vi "Ways to Win.vi"(11 "Race In":refnum<class "Race.lvclass">) -> (2 "Ways to win":u64, 3 "Race Out":refnum<class "Race.lvclass">)   [LabVIEW 2021, in "Race.lvclass"]
uses:
  Race.lvclass
  Race.lvclass/Race.ctl
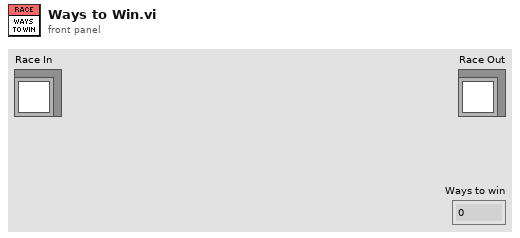
[diagram p1: front panel]
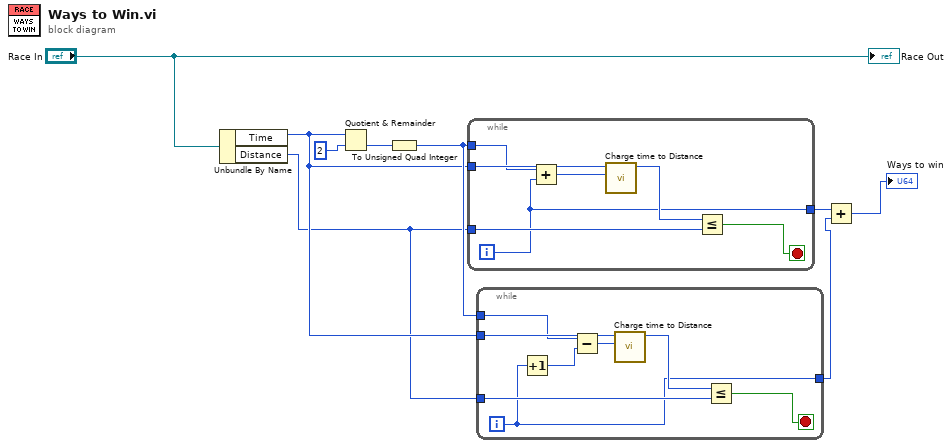
[diagram p0: block diagram]
diagram:
  n1 = Unbundle By Name("Race In") -> ("Time"=w4:u64, "Distance"=w3:u64)
  n2 = Quotient & Remainder(x=w4, y=u64 2) -> (floor(x/y)=w7:u64)  [unwired: 1 out]
  n3 = To Unsigned Quad Integer(1:w7) -> (0:w5:u64)
  n4 = while {
    tunnel: w4 -> [w16]
    tunnel: w5 -> [w15]
    tunnel: w3 -> [w12]
    tunnel: [w10] -> w6
    i -> [w10]
    stop <- w11 stop-if-true
    n5 = Add(x=w15, y=w10) -> (x+y=w14:u64)
    n6 = call "Charge time to Distance.vi"("Charge Time"=w14, "Raec Time"=w16) -> ("Distance"=w13:u64)  [unwired: 9 in]
    n7 = Less Or Equal?(x=w13, y=w12) -> (x <= y?=w11:bool)
  }
  n8 = while {
    tunnel: w4 -> [w24]
    tunnel: w5 -> [w23]
    tunnel: w3 -> [w20]
    tunnel: [w17] -> w2
    i -> [w17]
    stop <- w19 stop-if-true
    n9 = Increment(x=w17) -> (x+1=w18:i32)
    n10 = Subtract(x=w23, y=w18) -> (x-y=w22:u64)
    n11 = call "Charge time to Distance.vi"("Charge Time"=w22, "Raec Time"=w24) -> ("Distance"=w21:u64)  [unwired: 9 in]
    n12 = Less Or Equal?(x=w21, y=w20) -> (x <= y?=w19:bool)
  }
  n13 = Add(x=w6, y=w2) -> (x+y=→"Ways to win":i32)
  "Race Out" <- "Race In"
